vi "Null Broadcast Events--constant.vi"() -> (3 "Host Interpreter Broadcast Events":T1)   [LabVIEW 2021, in "Host Interpreter.lvlib"]
doc: "Returns the broadcast events cluster with null references for defining the event types in a Register For Events function.\n_____\nBased on DQMH Dev Tools: Project Template 7.1.2.1547."
uses:
  Host Interpreter.lvlib
  Broadcast Events--cluster.ctl
  Did Init Argument--cluster.ctl
  Status Updated Argument--cluster.ctl
  Error Reported Argument--cluster.ctl
  Stop Argument--cluster.ctl
  Get Module Execution Status Argument--cluster.ctl
  Connected Argument--cluster.ctl
  Update Target Connections Argument--cluster.ctl
  Disconnected Argument--cluster.ctl
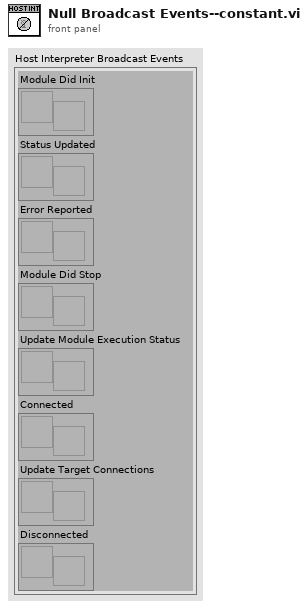
[diagram p1: front panel]
types:
  T1 = typedef "Host Interpreter.lvlib/Broadcast Events--cluster.ctl" = cluster{"Module Did Init":refnum<user-event>, "Status Updated":refnum<user-event>, "Error Reported":refnum<user-event>, "Module Did Stop":refnum<user-event>, "Update Module Execution Status":refnum<user-event>, "Connected":refnum<user-event>, "Update Target Connections":refnum<user-event>, "Disconnected":refnum<user-event>}
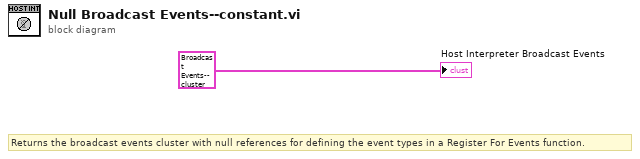
[diagram p0: block diagram]
diagram:
  # "Returns the broadcast events cluster with null references for defining the event types in a Register For Events function."
  "Host Interpreter Broadcast Events" <- T1 {"Module Did Init"=refnum, "Status Updated"=refnum, "Error Reported"=refnum, "Module Did Stop"=refnum, "Update Module Execution Status"=refnum, "Connected"=refnum, "Update Target Connections"=refnum, "Disconnected"=refnum} ("Broadcast Events")
